vi "LibCam_Close.vi"(8 "error in (no error)":errorcluster) -> (0 "error out":errorcluster)   [LabVIEW 2014, in "QwaveSys Raspberry Pi Library.lvlib"]
uses:
  QwaveSys Raspberry Pi Library.lvlib
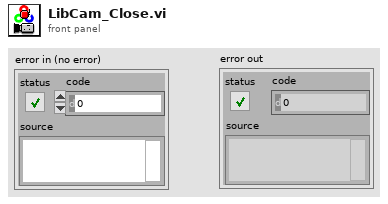
[diagram p1: front panel]
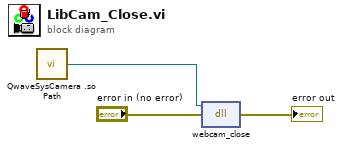
[diagram p0: block diagram]
diagram:
  n1 = call "QwaveSysCamera .so Path.vi"() -> ("QwaveSys .so Path"=w3:path)  [unwired: 5 in]
  n2 = dll-call lib="libcamera.so" fn="webcam_close"(path in=w3, error in="error in (no error)") -> (error out=→"error out":errorcluster)  [unwired: 2 in, 1 out]
